vi "UpdateSnakes.vi"(8 "error in (no error)":errorcluster, 10 "Engine in":refnum<class "Engine.lvclass">, 11 "SnakeGame in":refnum<class "SnakeGame.lvclass">) -> (0 "error out":errorcluster, 2 "Engine out":refnum<class "Engine.lvclass">, 3 "SnakeGame out":refnum<class "SnakeGame.lvclass">)   [LabVIEW 2019, in "RT_Game.lvlib" / "SnakeGame.lvclass"]
uses:
  SnakeGame.lvclass
  C:/Users/FreshBob/Dropbox/VIs/myRIO_GameConsole/RT/RT_Game/Game/Game.lvclass
  Engine/Engine.lvclass
  SnakeGame.lvclass/SnakeGame.ctl
  Engine/Engine.lvclass/Engine.ctl
  Snake/Snake.lvclass/Snake.ctl
  Game/Game.lvclass/Game.ctl
  Snake/Read Length.vi
  Game/Write Player1Score.vi
  Game/Write Player2Score.vi
  Snake/Snake.lvclass
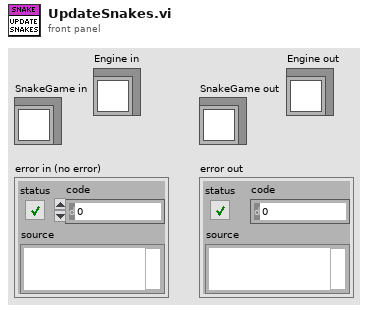
[diagram p1: front panel]
types:
  T1 = typedef "RT_Game.lvlib/Game.lvclass/Controls.ctl" = cluster{"Controls_1":T2, "Controls_2":cluster{"DirectionX":i8, "DirectionY":i8, "Button1":bool, "Button2":bool}, "SystemButton":bool}
  T2 = typedef "RT_Game.lvlib/Game.lvclass/ControlPlayer.ctl" = cluster{"DirectionX":i8, "DirectionY":i8, "Button1":bool, "Button2":bool}
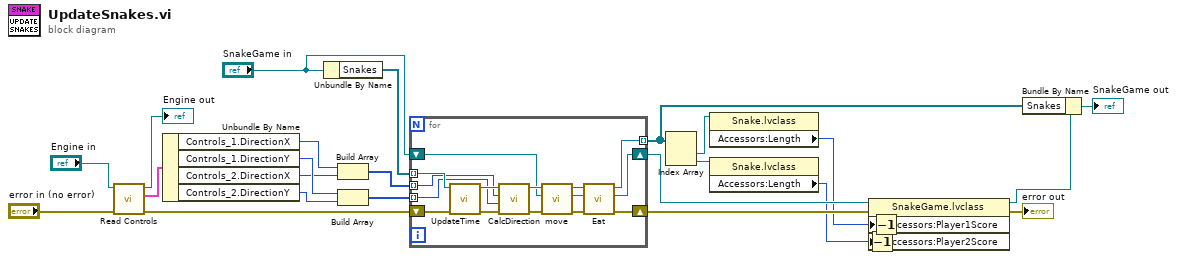
[diagram p0: block diagram]
diagram:
  n1 = call "Read Controls.vi"("error in (no error)"="error in (no error)", "Engine in"="Engine in") -> ("error out"=w14:errorcluster, "Controls"=w5:T1, "Engine out"=→"Engine out":refnum<class "Engine.lvclass">)  [unwired: 7 in]
  n2 = Unbundle By Name(w5) -> ("Controls_1.DirectionX"=w20:i8, "Controls_1.DirectionY"=w22:i8, "Controls_2.DirectionX"=w21:i8, "Controls_2.DirectionY"=w23:i8)
  n3 = Unbundle By Name("SnakeGame in") -> ("Snakes"=w17:refnum<class "Snake.lvclass">[])
  n4 = Build Array(w20, w21) -> (w24:i8[])
  n5 = Build Array(w22, w23) -> (w25:i8[])
  n6 = for {
    tunnel: w17 -> [w37] mode=indexing
    tunnel: [w29] -> w10 mode=indexing
    shift-right: [w31] -> w16
    shift-left: w14 -> [w40]
    tunnel: w24 -> [w33] mode=indexing
    tunnel: w25 -> [w32] mode=indexing
    shift-right: [w28] -> w12
    shift-left: "SnakeGame in" -> [w27]
    n7 = call "UpdateTime.vi"("error in (no error)"=w40, "Snake in"=w37) -> ("error out"=w38:errorcluster, "Snake out"=w35:refnum<class "Snake.lvclass">)  [unwired: 8 in]
    n8 = call "CalcDirection.vi"("error in (no error)"=w38, "DirectionY"=w32, "DirectionX"=w33, "Snake in"=w35) -> ("error out"=w36:errorcluster, "Snake out"=w34:refnum<class "Snake.lvclass">)  [unwired: 6 in]
    n9 = call "move.vi"("error in (no error)"=w36, "SnakeGame in"=w27, "Snake in"=w34) -> ("error out"=w39:errorcluster, "SnakeGame out"=w26:refnum<class "SnakeGame.lvclass">, "Snake out"=w30:refnum<class "Snake.lvclass">)  [unwired: 6 in]
    n10 = call "Eat.vi"("error in (no error)"=w39, "SnakeGame in"=w26, "Snake in"=w30) -> ("error out"=w31:errorcluster, "SnakeGame out"=w28:refnum<class "SnakeGame.lvclass">, "Snake out"=w29:refnum<class "Snake.lvclass">)  [unwired: 6 in]
  }
  n11 = Index Array(array=w10) -> (element #1=w9:refnum<class "Snake.lvclass">, element #2=w7:refnum<class "Snake.lvclass">)  [unwired: 2 in]
  n12 = property class="Snake.lvclass"(reference=w9) -> ("Accessors:Length"=w8:i16)  [unwired: 1 in, 2 out]
  n13 = property class="Snake.lvclass"(reference=w7) -> ("Accessors:Length"=w6:i16)  [unwired: 1 in, 2 out]
  n14 = Decrement(x=w6) -> (x-1=w1:i16)
  n15 = Decrement(x=w8) -> (x-1=w2:i16)
  n16 = property class="SnakeGame.lvclass"(reference=w12, error in=w16, "Accessors:Player1Score"=w2, "Accessors:Player2Score"=w1) -> (reference out=w11:refnum<class "SnakeGame.lvclass">, error out=→"error out":errorcluster)
  n17 = Bundle By Name(cluster=w11, "Snakes"=w10) -> (→"SnakeGame out":refnum<class "SnakeGame.lvclass">)
